vi "worksheet conditional format cell.vi"(7 "conditional_format":u32, 8 "error in (no error)":errorcluster, 9 "col":u16, 10 "row":u32, 11 "worksheet":u32) -> (0 "error out":errorcluster, 3 "function return":u32(ring))   [LabVIEW 2015, in "xlsxwriter.lvlib"]
doc: "lxw_error worksheet_conditional_format_cell(lxw_worksheet worksheet, lxw_row_t row, lxw_col_t col, unsigned long conditional_format);"
uses:
  xlsxwriter.lvlib
  xlsxwriter.dll
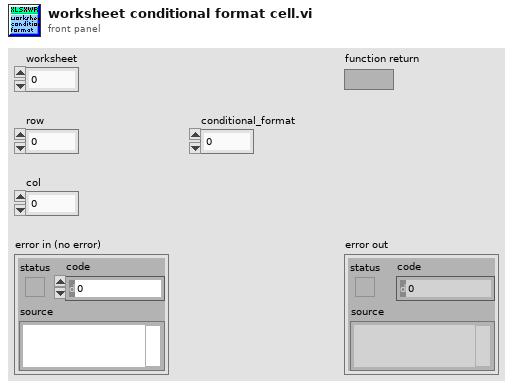
[diagram p1: front panel]
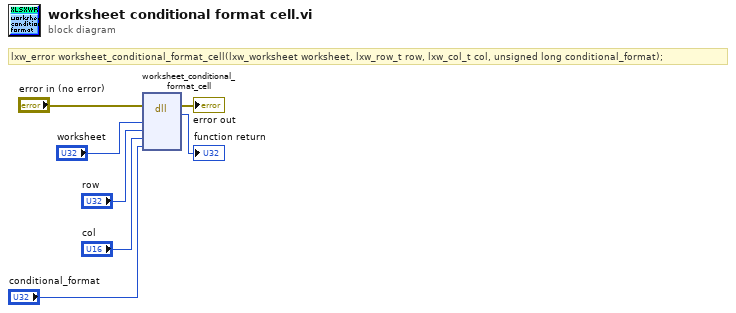
[diagram p0: block diagram]
diagram:
  # "lxw_error worksheet_conditional_format_cell(lxw_worksheet worksheet, lxw_row_t row, lxw_col_t col, unsigned long conditional_format);"
  n1 = dll-call lib="C:/Users/WDAGUtilityAccount/Desktop/lv_vis_added_cell/xlsxwriter.*" fn="worksheet_conditional_format_cell"(error in="error in (no error)", "worksheet"="worksheet", "row"="row", "col"="col", "conditional_format"="conditional_format") -> (error out=→"error out":errorcluster, →"function return":u32)  [unwired: 6 in, 1 out]
